vi "Main.vi"(11 "Module Admin":refnum<class "Delacor_lib_QMH_Module Admin.lvclass">) -> ()   [LabVIEW 2024, in "ProductControl.lvlib"]
doc: "This template is based off of the Queued Message Handler design pattern and the Queued Message Handler project template that ships with LabVIEW.\n\nThe main difference is that the queue is private to this module and communication between modules is performed via Broadcast and Request events.\n\nRequest events are wrapped in public API methods and are handled in the Event Handling Loop (EHL) of this VI. Any module can register for Broadcast events sent by this module. The EHL generates messages based on user interface actions.\n\nThe Message Handling Loop (MHL) processes messages generated by the EHL, or by other messages. The messages are string values, so new messages can be added easily to the Message Cases case structure in the MHL. Each message cluster can also provide an optional value for Message Data, which is a variant that can be converted to whatever message-specific data is required.\n_____\nBased on DQMH Dev Tools: Project Template 7.1.0.1503."
uses:
  ProductControl.lvlib
  <vilib>/Delacor/Delacor QMH/Libraries/Module Admin_class/Delacor_lib_QMH_Module Admin.lvclass
  Module Data--cluster.ctl
  Stop Argument--cluster.ctl
  <vilib>/Delacor/Delacor QMH/Libraries/Message Queue_class/Delacor_lib_QMH_Message Queue.lvclass/Delacor_lib_QMH_Message Queue.ctl
  <vilib>/Delacor/Delacor QMH/Libraries/Module Admin_class/Delacor_lib_QMH_Module Admin.lvclass/Delacor_lib_QMH_Module Admin.ctl
  Draw FP in Subpanel Argument--cluster.ctl
  Remove From Subpanel Argument--cluster.ctl
  Vender Producto Argument--cluster.ctl
  <vilib>/Delacor/Delacor QMH/Libraries/Message Queue_class/Delacor_lib_QMH_Enqueue Message (Single).vi
  <vilib>/Delacor/Delacor QMH/Libraries/Module Admin_class/Delacor_lib_QMH_Get External Launch.vi
  <vilib>/Delacor/Delacor QMH/Libraries/Message Queue_class/Delacor_lib_QMH_Message Queue.lvclass
panel:
  in  "Productos":i32(listbox)
  out "error out":errorcluster
  out "Status":string
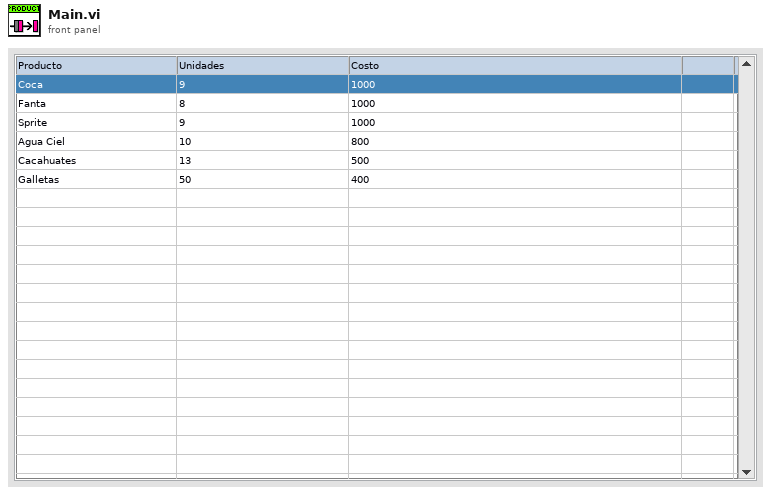
[diagram p1: front panel]
types:
  T1 = typedef "ProductControl.lvlib/Request Events--cluster.ctl" = cluster{"Stop Module":refnum<user-event>, "Show Panel":refnum<user-event>, "Hide Panel":refnum<user-event>, "Get Module Execution Status":refnum<user-event>, "Show Diagram":refnum<user-event>, "Draw FP in Subpanel":refnum<user-event>, "Remove From Subpanel":refnum<user-event>, "Vender Producto":refnum<user-event>}
  T2 = typedef "ProductControl.lvlib/Module Data--cluster.ctl" = cluster{"Status":string, "Sub Panel":refnum<vi>}
  T3 = enum32{"invalid lock state", "Not Locked", "Locked (No Password)", "Password-protected"}
  T4 = typedef "ProductControl.lvlib/Stop Argument--cluster.ctl" = cluster{"Origin":string, "Exit via Stop Module Req?":bool, "Wait for Module to stop?":bool}
  T5 = typedef "ProductControl.lvlib/Draw FP in Subpanel Argument--cluster.ctl" = cluster{"Sub Panel":refnum<vi>}
  T6 = typedef "ProductControl.lvlib/Remove From Subpanel Argument--cluster.ctl" = cluster{"Boolean":bool}
  T7 = typedef "ProductControl.lvlib/Vender Producto Argument--cluster.ctl" = cluster{"Nombre Producto":string}
  T8 = enum32{"Invalid", "Standard", "Closed", "Hidden", "Minimized", "Maximized"}
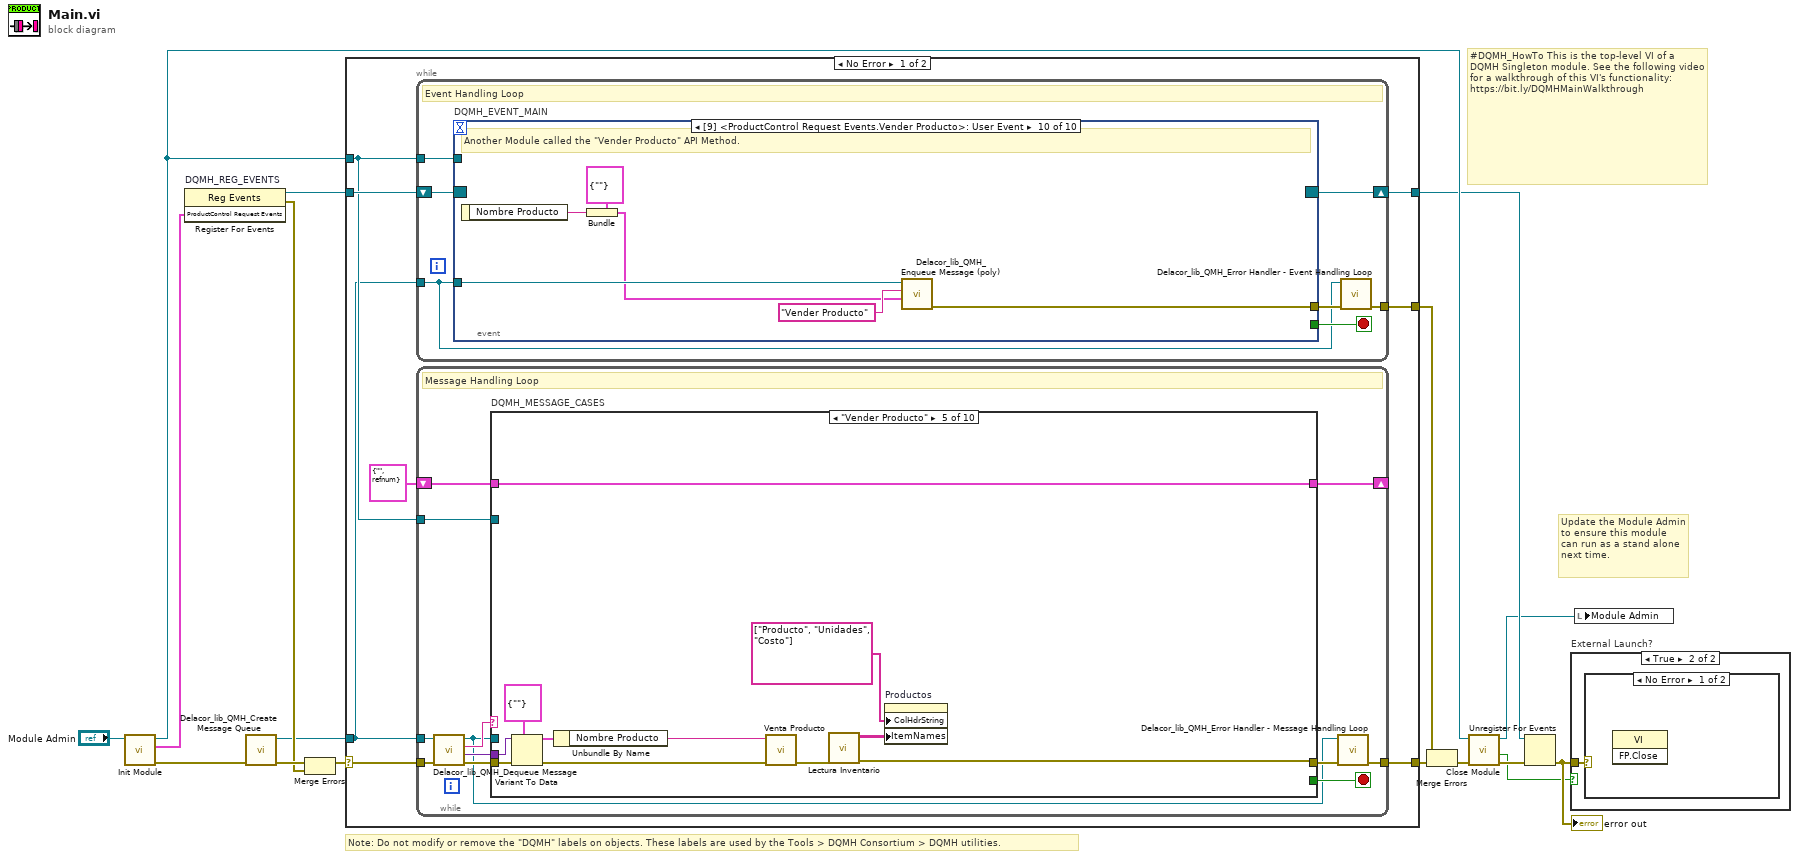
[diagram p0: block diagram]
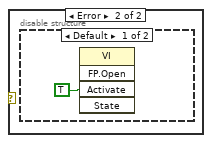
[diagram p3: hidden frame]
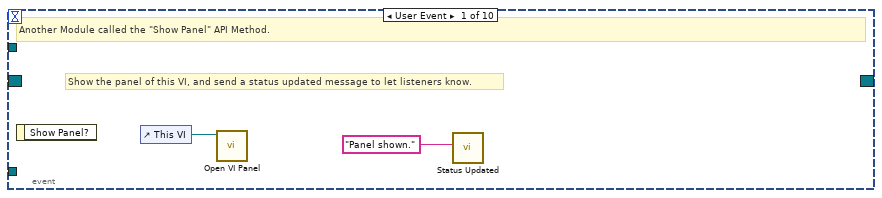
[diagram p5: hidden frame]
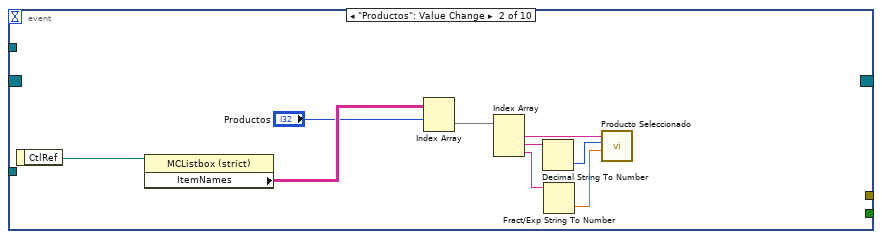
[diagram p6: hidden frame]
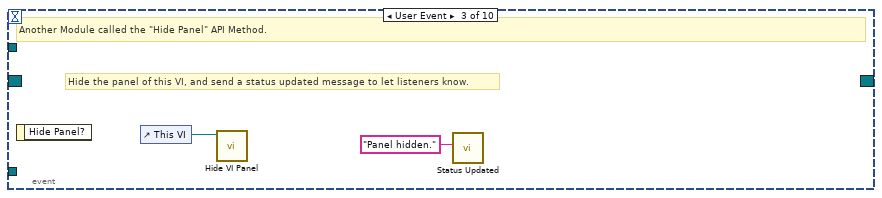
[diagram p7: hidden frame]
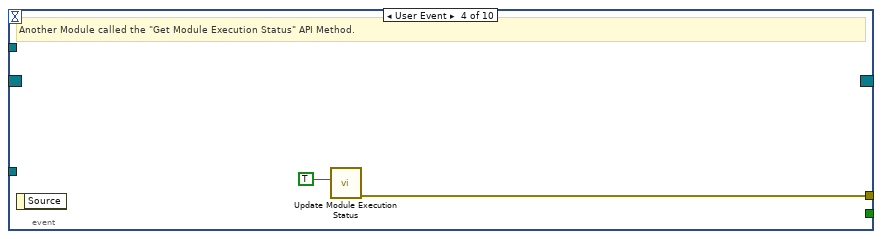
[diagram p8: hidden frame]
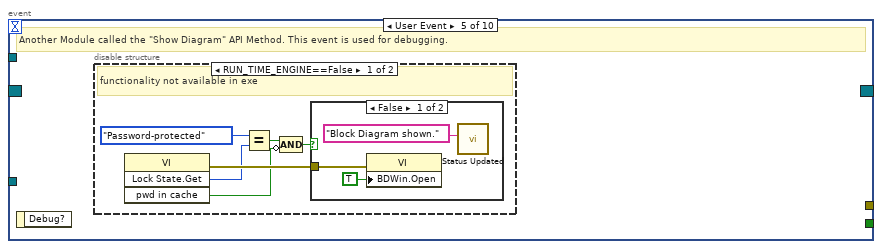
[diagram p9: hidden frame]
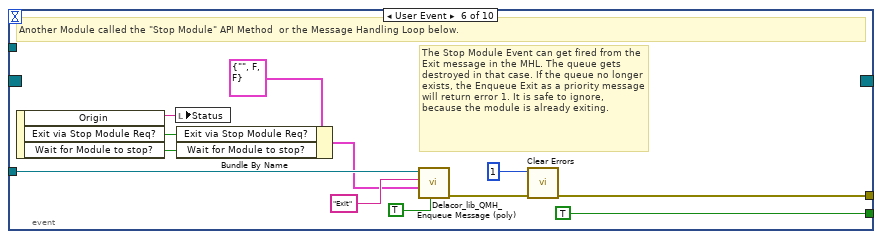
[diagram p12: hidden frame]
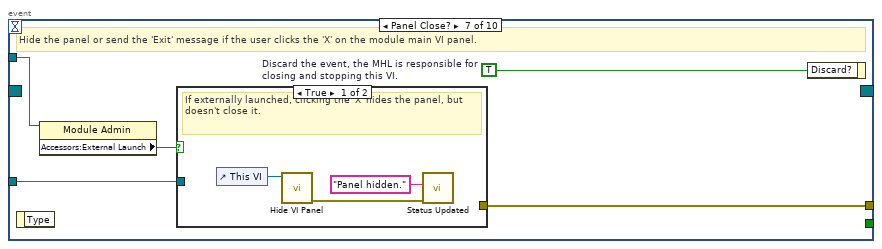
[diagram p13: hidden frame]
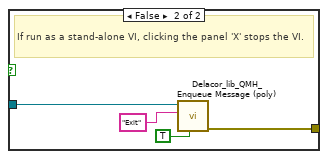
[diagram p14: hidden frame]
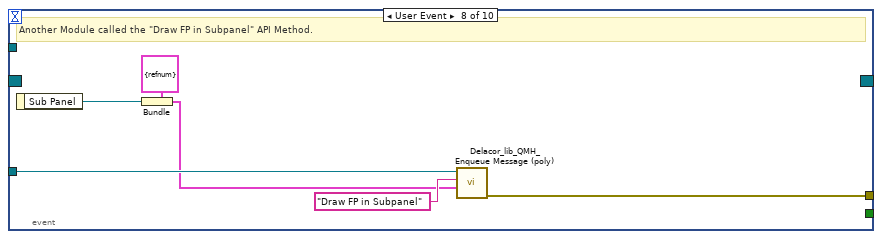
[diagram p15: hidden frame]
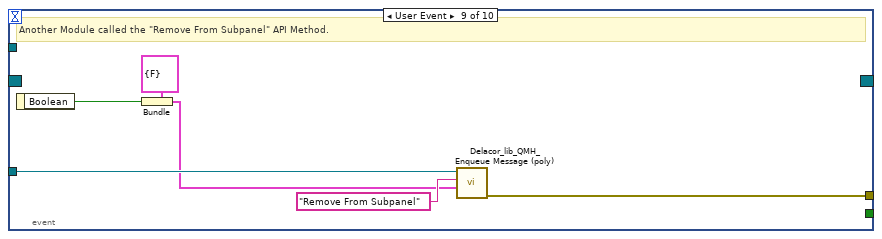
[diagram p16: hidden frame]
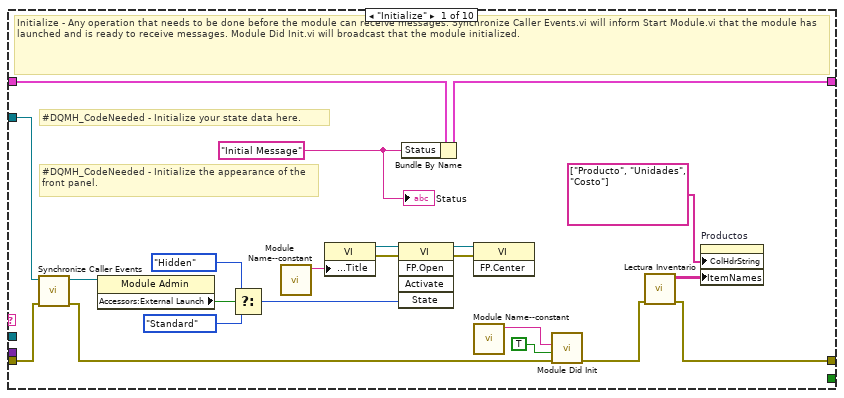
[diagram p17: hidden frame]
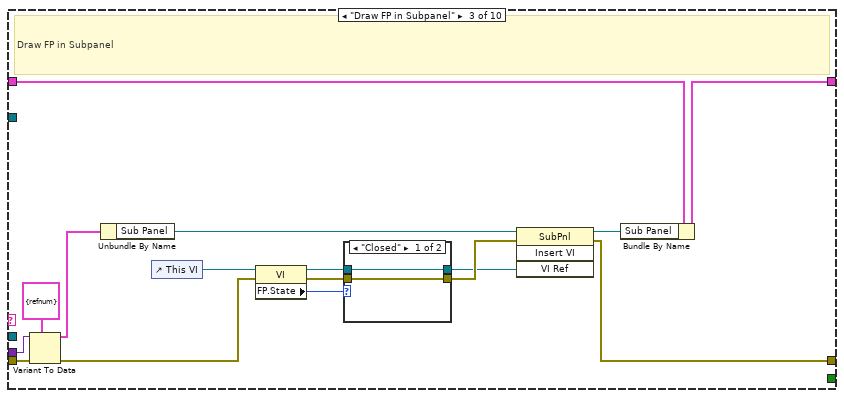
[diagram p19: hidden frame]
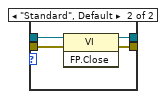
[diagram p20: hidden frame]
diagram:
  # "#DQMH_HowTo This is the top-level VI of a DQMH Singleton module. See the following video for a walkthrough of this VI's functionality: https://bit.ly/DQMHMainWalkthrough"
  # "Note: Do not modify or remove the \"DQMH\" labels on objects. These labels are used by the Tools > DQMH Consortium > DQMH utilities."
  # "Update the Module Admin to ensure this module can run as a stand alone next time."
  n1 = call "Init Module.vi"("Singleton Module Admin in"="Module Admin") -> ("error out"=w16:errorcluster, "ProductControl Request Events"=w5:T1, "Singleton Module Admin out"=w8:refnum<class "Delacor_lib_QMH_Module Admin.lvclass">)  [unwired: 8 in]
  n2 = register-events "DQMH_REG_EVENTS"(w5) -> (reference out=w6:refnum<event-registration>, error out=w9:errorcluster)  [unwired: 2 in]
  n3 = call <vilib>:"Delacor_lib_QMH_Create Message Queue.vi"("error in"=w16) -> ("error out"=w11:errorcluster, "Message Queue"=w4:refnum<class "Delacor_lib_QMH_Message Queue.lvclass">)  [unwired: 9 in]
  n4 = Merge Errors(w11, w9) -> (w10:errorcluster)
  n5 = case shown="No Error" w10 {
    selector: w10 -> [w23 w241]
    tunnel: [w25 w240] -> w17
    tunnel: [w22 w239] -> w7
    tunnel: w6 -> [w20 w239]
    tunnel: w4 -> [w18 w234]
    tunnel: [w24 _] -> w14
    tunnel: w8 -> [w19 w235]
    frame No Error {
      n6 = while {
        tunnel: w18 -> [w26]
        shift-right: [w29] -> w22
        shift-left: w20 -> [w30]
        tunnel: [w31] -> w24
        tunnel: w19 -> [w27]
        stop <- w28 stop-if-true
        # "Event Handling Loop"
        n7 = event "DQMH_EVENT_MAIN" shown="[9] <ProductControl Request Events.Vender Producto>: User Event" {
          selector: w30 -> [_ _ _ _ _ _ _ _ _ _]
          dyn-events: [_ _ _ _ _ _ _ _ _ _] -> w29
          timeout: _ -> [_ _ _ _ _ _ _ _ _ _]
          tunnel: [_ _ _ _ _ TRUE ("Discard?") _ _ _ _] -> w28
          tunnel: w26 -> [_ _ _ _ _ w64 w71 w85 w91 w97]
          tunnel: [_ _ _ w47 _ w67 w73 w86 w92 w98] -> w32
          tunnel: w27 -> [_ _ _ _ _ _ w70 _ _ _]
          event User Event {
            # "Show the panel of this VI, and send a status updated message to let listeners know."
            # "Another Module called the \"Show Panel\" API Method."
            n8 = event-data() -> ()  [unwired: 1 in, 1 out]
            n9 = control-ref of="This VI"() -> (w34:refnum<vi>)
            n10 = call "Open VI Panel.vi"("VI"=w34) -> ()  [unwired: 10 in, 1 out]
            n11 = call "Status Updated.vi"("Status"="Panel shown." ("format string")) -> ()  [unwired: 10 in, 1 out]
          }
          event "Productos": Value Change {
            n12 = event-data() -> ("CtlRef"=w43:refnum<vi>)  [unwired: 1 in]
            n13 = property class="MCListbox (strict)"(reference=w43) -> ("ItemNames"=w42:string[][])  [unwired: 1 in, 2 out]
            n14 = Index Array(array=w42, index (row)="Productos") -> (element=w40:string[])  [unwired: 1 in]
            n15 = Index Array(array=w40) -> (element #1=w39:string, element #2=w38:string, element #3=w36:string)  [unwired: 3 in]
            n16 = Decimal String To Number(string=w38) -> (number=w37:i32)  [unwired: 2 in, 1 out]
            n17 = Fract/Exp String To Number(string=w36) -> (number=w35:dbl)  [unwired: 3 in, 1 out]
            n18 = call "Producto Seleccionado.vi"("Costo"=w35, "Unidades"=w37, "Nombre Producto"=w39) -> ()  [unwired: 8 in, 1 out]
          }
          event User Event {
            # "Hide the panel of this VI, and send a status updated message to let listeners know."
            # "Another Module called the \"Hide Panel\" API Method."
            n19 = event-data() -> ()  [unwired: 1 in, 1 out]
            n20 = control-ref of="This VI"() -> (w45:refnum<vi>)
            n21 = call "Hide VI Panel.vi"("VI"=w45) -> ()  [unwired: 10 in, 1 out]
            n22 = call "Status Updated.vi"("Status"="Panel hidden." ("format string")) -> ()  [unwired: 10 in, 1 out]
          }
          event User Event {
            # "Another Module called the \"Get Module Execution Status\" API Method."
            n23 = event-data() -> ()  [unwired: 1 in, 1 out]
            n24 = call "Update Module Execution Status.vi"("Running?"=TRUE) -> ("error out"=w47:errorcluster)  [unwired: 10 in]
          }
          event User Event {
            # "Another Module called the \"Show Diagram\" API Method. This event is used for debugging."
            n25 = event-data() -> ()  [unwired: 1 in, 1 out]
            n26 = disable-structure shown="RUN_TIME_ENGINE==False" {
              frame condition #0 (active) {
                # "functionality not available in exe"
                n27 = invoke on="Invoke Node" class="VI" method="Lock State.Get"() -> (error out=w53:errorcluster, "Get Lock State"=w52:T3, "pwd in cache"=w49:bool)  [unwired: 4 in, 1 out]
                n28 = Equal?(x=T3."Password-protected", y=w52) -> (x = y?=w50:bool)
                n29 = Compound Arithmetic op=AND(w50, invert w49) -> (w48:bool)
                n30 = case shown="False" w48 {
                  tunnel: w53 -> [w56 _]
                  frame False {
                    n31 = property on="Property Node" class="VI"(error in=w56, "BDWin.Open"=TRUE ("Block Diagram Window:Open")) -> ()  [unwired: 1 in, 2 out]
                    n32 = call "Status Updated.vi"("Status"="Block Diagram shown." ("format string")) -> ()  [unwired: 10 in, 1 out]
                  }
                  frame True {
                    # "Password-protected VI, and the password is not in the cache. Do not show the diagram."
                  }
                }
              }
              frame condition #1 {
              }
            }
          }
          event User Event {
            # "The Stop Module Event can get fired from the Exit message in the MHL. The queue gets destroyed in that case. If the queue no longer exists, the Enqueue Exit as a priority message will return error 1. It is safe to ignore, because the module is already exiting."
            # "Another Module called the \"Stop Module\" API Method  or the Message Handling Loop below."
            n33 = event-data() -> ("Origin"=w63:string, "Exit via Stop Module Req?"=w59:bool, "Wait for Module to stop?"=w58:bool)  [unwired: 1 in]
            n34 = local write "Status"(w63) -> ()
            n35 = Bundle By Name(cluster=T4 {"Origin"="", "Exit via Stop Module Req?"=FALSE, "Wait for Module to stop?"=FALSE} ("Stop Argument"), "Exit via Stop Module Req?"=w59, "Wait for Module to stop?"=w58) -> (w57:T4)
            n36 = call-poly <vilib>:"Delacor_lib_QMH_Enqueue Message (poly).vi"("Priority Message? (F)"=TRUE, "Message Data"=w57, "Message"="Exit", "Message Queue in"=w64) -> ("error out"=w68:errorcluster)  [unwired: 6 in, 1 out]
            n37 = call <vilib>:"Clear Errors.vi"("error in (no error)"=w68, "specific error code to clear (0: all)"=1) -> ("error out"=w67:errorcluster)  [unwired: 4 in, 1 out]
          }
          event Panel Close? {
            w72 = TRUE  # Discard the event, the MHL is responsible for closing and stopping this VI.
            # "Hide the panel or send the 'Exit' message if the user clicks the 'X' on the module main VI panel."
            n38 = event-data() -> ()  [unwired: 1 in, 1 out]
            n39 = property on="Property Node" class="Module Admin"(reference=w70) -> ("Accessors:External Launch"=w69:bool)  [unwired: 1 in, 2 out]
            n40 = case shown="True" w69 {
              tunnel: w71 -> [_ w79]
              tunnel: [_ w80] -> w73
              frame True {
                # "If externally launched, clicking the 'X' hides the panel, but doesn't close it."
                n41 = control-ref of="This VI"() -> (w75:refnum<vi>)
                n42 = call "Hide VI Panel.vi"("VI"=w75) -> ("error out"=w76:errorcluster)  [unwired: 10 in]
                n43 = call "Status Updated.vi"("error in"=w76, "Status"="Panel hidden." ("format string")) -> ()  [unwired: 9 in, 1 out]
              }
              frame False {
                # "If run as a stand-alone VI, clicking the panel 'X' stops the VI."
                n44 = call-poly <vilib>:"Delacor_lib_QMH_Enqueue Message (poly).vi"("Priority Message? (F)"=TRUE, "Message"="Exit", "Message Queue in"=w79) -> ("error out"=w80:errorcluster)  [unwired: 7 in, 1 out]
              }
            }
            n45 = event-data ("Event Filter Node")("Discard?"=w72) -> ()  [unwired: 1 in, 1 out]
          }
          event User Event {
            # "Another Module called the \"Draw FP in Subpanel\" API Method."
            n46 = event-data() -> ("Sub Panel"=w81:refnum<vi>)  [unwired: 1 in]
            n47 = Bundle(cluster=T5 {"Sub Panel"=refnum} ("Draw FP in Subpanel Argument"), "Sub Panel"=w81) -> (w82:T5)
            n48 = call-poly <vilib>:"Delacor_lib_QMH_Enqueue Message (poly).vi"("Message Data"=w82, "Message"="Draw FP in Subpanel", "Message Queue in"=w85) -> ("error out"=w86:errorcluster)  [unwired: 7 in, 1 out]
          }
          event User Event {
            # "Another Module called the \"Remove From Subpanel\" API Method."
            n49 = event-data() -> ("Boolean"=w87:bool)  [unwired: 1 in]
            n50 = Bundle(cluster=T6 {"Boolean"=FALSE} ("Remove From Subpanel Argument"), "Boolean"=w87) -> (w88:T6)
            n51 = call-poly <vilib>:"Delacor_lib_QMH_Enqueue Message (poly).vi"("Message Data"=w88, "Message"="Remove From Subpanel", "Message Queue in"=w91) -> ("error out"=w92:errorcluster)  [unwired: 7 in, 1 out]
          }
          event User Event {
            # "Another Module called the \"Vender Producto\" API Method."
            n52 = event-data() -> ("Nombre Producto"=w93:string)  [unwired: 1 in]
            n53 = Bundle(cluster=T7 {"Nombre Producto"=""} ("Vender Producto Argument"), "Nombre Producto"=w93) -> (w94:T7)
            n54 = call-poly <vilib>:"Delacor_lib_QMH_Enqueue Message (poly).vi"("Message Data"=w94, "Message"="Vender Producto", "Message Queue in"=w97) -> ("error out"=w98:errorcluster)  [unwired: 7 in, 1 out]
          }
        }
        n55 = call-dynamic "Delacor_lib_QMH_Error Handler - Event Handling Loop.vi"("error in"=w32, "Message Queue in"=w26) -> ("dup error in"=w31:errorcluster)  [unwired: 8 in, 1 out]
      }
      n56 = while {
        tunnel: w18 -> [w99]
        shift-right: [w105] -> _
        shift-left: T2 {"Status"="", "Sub Panel"=refnum} ("Data Cluster") -> [w106]
        tunnel: w23 -> [w110]
        tunnel: [w108] -> w25
        tunnel: w19 -> [w101]
        stop <- w104 stop-if-true
        # "Message Handling Loop"
        n57 = call-dynamic "Delacor_lib_QMH_Dequeue Message.vi"("error in"=w110, "Message Queue in"=w99) -> ("error out"=w109:errorcluster, "Message Data"=w102:variant, "Message"=w103:string, "Message Queue out"=w100:refnum<class "Delacor_lib_QMH_Message Queue.lvclass">)  [unwired: 6 in]
        n58 = case "DQMH_MESSAGE_CASES" shown="\"Vender Producto\"" w103 {
          selector: w103 -> [_ _ _ _ _ _ _ _ _ w229]
          tunnel: w100 -> [_ _ _ _ _ _ _ w193 w217 _]
          tunnel: w109 -> [w130 w134 w150 w168 w185 w188 w190 w201 w223 w232]
          tunnel: [w127 w134 w149 w166 w182 w187 w190 w197 w218 w233] -> w107
          tunnel: w106 -> [w118 w133 w145 w162 w181 w186 w189 w195 w209 w230]
          tunnel: [w117 w133 w141 w159 w181 w186 w189 w195 w209 w230] -> w105
          tunnel: [_ _ _ _ _ _ _ _ w216 _] -> w104
          tunnel: w102 -> [_ _ w144 w165 w180 _ _ w194 w215 _]
          tunnel: w101 -> [w119 _ _ _ _ _ _ w192 w210 _]
          frame "Initialize" {
            w113 = "Initial Message" ("Initial Message")
            # "#DQMH_CodeNeeded - Initialize the appearance of the front panel."
            # "#DQMH_CodeNeeded - Initialize your state data here."
            # "Initialize - Any operation that needs to be done before the module can receive messages. Synchronize Caller Events.vi will inform Start Module.vi that the module has launched and is ready to receive messages. Module Did Init.vi will broadcast that the module initialized."
            n59 = call "Synchronize Caller Events.vi"("error in"=w130, "Singleton Module Admin in"=w119) -> ("error out"=w129:errorcluster, "Singleton Module Admin out"=w114:refnum<class "Delacor_lib_QMH_Module Admin.lvclass">)  [unwired: 8 in]
            n60 = property on="Property Node" class="Module Admin"(reference=w114) -> ("Accessors:External Launch"=w123:bool)  [unwired: 1 in, 2 out]
            n61 = Select(t=T8."Hidden" ("State"), s=w123, f=T8."Standard" ("State")) -> (s? t:f=w120:T8)
            n62 = call "Module Name--constant.vi"() -> ("Module Name"=w126:string)  [unwired: 11 in]
            n63 = property on="Property Node" class="VI"("Front Panel.Title"=w126) -> (reference out=w125:refnum<vi>, error out=w132:errorcluster)  [unwired: 2 in]
            n64 = invoke on="Invoke Node" class="VI" method="FP.Open"(reference=w125, error in=w132, "State"=w120) -> (reference out=w124:refnum<vi>, error out=w131:errorcluster)  [unwired: 2 in, 3 out]
            n65 = Bundle By Name(cluster=w118, "Status"=w113) -> (w117:T2)
            n66 = invoke on="Invoke Node" class="VI" method="FP.Center"(reference=w124, error in=w131) -> ()  [unwired: 1 in, 3 out]
            n67 = call "Module Name--constant.vi"() -> ("Module Name"=w115:string)  [unwired: 11 in]
            n68 = call "Module Did Init.vi"("error in"=w129, "Initialized?"=TRUE, "Origin"=w115) -> ("error out"=w128:errorcluster)  [unwired: 8 in]
            n69 = call "Lectura Inventario.vi"("error in"=w128) -> ("error out"=w127:errorcluster, "Inventario"=w112:string[][])  [unwired: 9 in]
            n70 = property on="Productos" class="MCListbox (strict)"("ColHdrString"=string[] ["Producto", "Unidades", "Costo"] ("Column Header Strings[]"), "ItemNames"=w112) -> ()  [unwired: 2 in, 2 out]
            "Status" <- w113
          }
          frame "---Module Specific---" {
            # "Separator -- The following cases handle messages specific to this Module."
          }
          frame "Draw FP in Subpanel" {
            # "Draw FP in Subpanel"
            n71 = Variant To Data(error in=w150, type=T5 {"Sub Panel"=refnum} ("Draw FP in Subpanel Argument"), Variant=w144) -> (data=w142:T5, error out=w148:errorcluster)
            n72 = Unbundle By Name(w142) -> ("Sub Panel"=w140:refnum<vi>)
            n73 = control-ref of="This VI"() -> (w137:refnum<vi>)
            n74 = property class="VI"(reference=w137, error in=w148) -> (reference out=w136:refnum<vi>, error out=w146:errorcluster, "FP.State"=w135:T8)
            n75 = case shown="\"Closed\"" w135 {
              tunnel: [w151 w154] -> w138
              tunnel: [w152 w156] -> w147
              tunnel: w146 -> [w152 w155]
              tunnel: w136 -> [w151 w153]
              frame "Closed" {
              }
              frame "Standard", Default {
                n76 = invoke class="VI" method="FP.Close"(reference=w153, error in=w155) -> (reference out=w154:refnum<vi>, error out=w156:errorcluster)  [unwired: 1 in, 1 out]
              }
            }
            n77 = invoke class="SubPnl" method="Insert VI"(reference=w140, error in=w147, "VI Ref"=w138) -> (reference out=w139:refnum<vi>, error out=w149:errorcluster)  [unwired: 1 in, 2 out]
            n78 = Bundle By Name(cluster=w145, "Sub Panel"=w139) -> (w141:T2)
          }
          frame "Remove From Subpanel" {
            # "Remove From Subpanel"
            n79 = Variant To Data(error in=w168, type=T6 {"Boolean"=FALSE} ("Remove From Subpanel Argument"), Variant=w165) -> (data=w163:T6, error out=w167:errorcluster)
            n80 = Unbundle By Name(w163) -> ()  [unwired: 1 out]
            n81 = Unbundle By Name(w162) -> ("Sub Panel"=w161:refnum<vi>)
            n82 = Not A Number/Path/Refnum?(number/path/refnum=w161) -> (NaN/Path/Refnum?=w160:bool)
            n83 = case shown="True" w160 {
              tunnel: w167 -> [w172 w174]
              tunnel: [w171 w174] -> w166
              tunnel: w161 -> [w170 _]
              tunnel: ["Module Removed from Subpanel" "This module has not been inserted into the subpanel"] -> w157
              frame False {
                n84 = invoke class="SubPnl" method="Remove VI"(reference=w170, error in=w172) -> (error out=w171:errorcluster)  [unwired: 1 in, 2 out]
              }
              frame True {
              }
            }
            n85 = Bundle By Name(cluster=w162, "Sub Panel"=refnum<vi> refnum) -> (w159:T2)
            n86 = call "Status Updated.vi"("Status"=w157) -> ()  [unwired: 10 in, 1 out]
          }
          frame "Vender Producto" {
            n87 = Variant To Data(error in=w185, type=T7 {"Nombre Producto"=""} ("Vender Producto Argument"), Variant=w180) -> (data=w178:T7, error out=w184:errorcluster)
            n88 = Unbundle By Name(w178) -> ("Nombre Producto"=w177:string)
            n89 = call "Venta Producto.vi"("error in"=w184, "Nombre Producto"=w177) -> ("error out"=w183:errorcluster)  [unwired: 9 in]
            n90 = call "Lectura Inventario.vi"("error in"=w183) -> ("error out"=w182:errorcluster, "Inventario"=w176:string[][])  [unwired: 9 in]
            n91 = property on="Productos" class="MCListbox (strict)"("ColHdrString"=string[] ["Producto", "Unidades", "Costo"] ("Column Header Strings[]"), "ItemNames"=w176) -> ()  [unwired: 2 in, 2 out]
          }
          frame "---Copy This Frame---" {
            # "Duplicate this frame when creating new messages.  Change this comment in the duplicated frame to describe this message."
            n92 = Merge Errors(w188) -> (w187:errorcluster)
          }
          frame "---Exit and Error Handling---" {
            # "Separator - The following cases handle errors and exit messages."
          }
          frame "Error" {
            # "#DQMH_CodeRecommended - If the module is running in standalone mode (External Launch = FALSE), this code will pop up an error dialog and call the 'Exit' message if an error occurs. Add more fine-grained error management here."
            # "Error - Check the error message data and respond accordingly. This message is sent by the \"Error Handler\" VIs at the end of each loop in this application."
            n93 = property on="Property Node" class="Module Admin"(reference=w192) -> ("Accessors:External Launch"=w191:bool)  [unwired: 1 in, 2 out]
            n94 = Variant To Data(error in=w201, type=errorcluster {"status"=FALSE, "code"=0, "source"=""} ("error constant"), Variant=w194) -> (data=w196:errorcluster, error out=w199:errorcluster)
            n95 = local write "error out"(w196) -> ()
            n96 = call "Error Reported.vi"("Error"=w196) -> ()  [unwired: 10 in, 1 out]
            n97 = case shown="False" w191 {
              tunnel: [w206 _] -> w198
              tunnel: w193 -> [w204 _]
              tunnel: w196 -> [w205 _]
              frame False {
                n98 = disable-structure shown="Default" {
                  disable-tunnel: w205 -> [w207 _]
                  frame condition #0 (active) {
                    # "If the module is running standalone, then pop up an error dialog and call the \"Exit\" message."
                    n99 = call <vilib>:"Simple Error Handler.vi"("error in (no error)"=w207) -> ()  [unwired: 4 in, 5 out]
                  }
                  frame condition #1 {
                    # "To prevent the Simple Error Handler VI from being loaded (e.g. when deploying to a Real-Time target), add the Conditional Disable Symbol \"DQMH_Disable_SEH\" to your project and set it to TRUE."
                  }
                }
                n100 = call-poly <vilib>:"Delacor_lib_QMH_Enqueue Message (poly).vi"("Priority Message? (F)"=TRUE, "Message"="Exit", "Message Queue in"=w204) -> ("error out"=w206:errorcluster)  [unwired: 7 in, 1 out]
              }
              frame True {
                # "If the module was launched externally, calling the Error Reported broadcast VI is the only action performed by the \"Error\" message. The module's caller can then process the error appropriately."
              }
            }
            n101 = Merge Errors(w199, w198) -> (w197:errorcluster)
          }
          frame "Exit" {
            w214 = 91  # 91: not all Exit messages will have an argument
            w216 = TRUE  # Stop the VI
            # "Release the message queue reference"
            # "#DQMH_CodeNeeded - Add any required cleanup code here."
            # "Exit - Exit the application."
            n102 = Variant To Data(error in=w223, type=T4 {"Origin"="", "Exit via Stop Module Req?"=FALSE, "Wait for Module to stop?"=FALSE} ("Stop Argument"), Variant=w215) -> (data=w212:T4, error out=w220:errorcluster)
            n103 = call <vilib>:"Clear Errors.vi"("error in (no error)"=w220, "specific error code to clear (0: all)"=w214) -> ("error out"=w222:errorcluster)  [unwired: 4 in, 1 out]
            n104 = control-ref of="This VI"() -> (w211:refnum<vi>)
            n105 = call-dynamic "Delacor_lib_QMH_Release Message Queue.vi"("error in"=w222, "Message Queue"=w217) -> ("error out"=w221:errorcluster)  [unwired: 9 in]
            n106 = call "Handle Exit.vi"("Stop Argument"=w212, "Admin in"=w210, "VI reference"=w211) -> ("error out"=w219:errorcluster)  [unwired: 7 in, 1 out]
            n107 = Merge Errors(w221, w219) -> (w218:errorcluster)
            n108 = Unbundle By Name(w209) -> ("Sub Panel"=w208:refnum<vi>)
            n109 = call "Error Reported.vi"("Error"=w218) -> ()  [unwired: 10 in, 1 out]
            n110 = invoke class="SubPnl" method="Remove VI"(reference=w208) -> ()  [unwired: 2 in, 3 out]
          }
          frame Default {
            # "'Default' case only runs if there is a message that isn't defined in any of the other cases.  Output a programming error."
            n111 = call "Module Name--constant.vi"() -> ("Module Name"=w228:string)  [unwired: 11 in]
            n112 = Format Into String(format string="The invalid message string \"%s\" was received in the Message Handling Loop for module \"%s\".", w229, w228) -> (resulting string=w224:string)  [unwired: 2 in, 1 out]
            n113 = call <vilib>:"Error Cluster From Error Code.vi"("show call chain? (False)"=TRUE, "error message (\"\")"=w224, "error code (0)"=1) -> ("error out"=w231:errorcluster)  [unwired: 6 in]
            n114 = Merge Errors(w232, w231) -> (w233:errorcluster)
          }
        }
        n115 = call-dynamic "Delacor_lib_QMH_Error Handler - Message Handling Loop.vi"("error in"=w107, "Message Queue in"=w100) -> ("dup error in"=w108:errorcluster)  [unwired: 8 in, 1 out]
      }
    }
    frame Error {
      # "Synchronize Caller Events.vi will inform Start Module.vi that the module has launched and will let the code calling Start Module.vi register for broadcasts and would permit the caller receive the broadcast that an error occurred at launch time."
      n116 = call-dynamic "Delacor_lib_QMH_Release Message Queue.vi"("error in"=w241, "Message Queue"=w234) -> ("error out"=w240:errorcluster)  [unwired: 9 in]
      n117 = call "Synchronize Caller Events.vi"("Singleton Module Admin in"=w235) -> ("error out"=w242:errorcluster)  [unwired: 9 in, 1 out]
      n118 = call "Module Name--constant.vi"() -> ("Module Name"=w238:string)  [unwired: 11 in]
      n119 = Format Into String(format string="An error occurred during initialization. %s is no longer running.", w238) -> (resulting string=w236:string)  [unwired: 2 in, 1 out]
      n120 = Merge Errors(w240, w242) -> (w243:errorcluster)
      n121 = call "Error Reported.vi"("Additional Information"=w236, "Error"=w243) -> ()  [unwired: 9 in, 1 out]
    }
  }
  n122 = Merge Errors(w14, w17) -> (w13:errorcluster)
  n123 = call "Close Module.vi"("error in"=w13, "Module Admin in"=w8) -> ("error out"=w15:errorcluster, "External Launch"=w1:bool, "Module Admin out"=w2:refnum<class "Delacor_lib_QMH_Module Admin.lvclass">)  [unwired: 7 in]
  n124 = Unregister For Events(event registration refnum=w7, error in=w15) -> (error out=w12:errorcluster)
  "error out" <- w12
  n125 = case "External Launch?" shown="True" w1 {
    tunnel: w12 -> [_ w244]
    frame False {
    }
    frame True {
      n126 = case shown="No Error" w244 {
        frame No Error {
          n127 = invoke on="Invoke Node" class="VI" method="FP.Close"() -> ()  [unwired: 3 in, 3 out]
        }
        frame Error {
          n128 = disable-structure shown="Default" {
            frame condition #0 (active) {
              n129 = invoke class="VI" method="FP.Open"("Activate"=TRUE ("Activate?")) -> ()  [unwired: 4 in, 5 out]
            }
            frame condition #1 {
              # "Don't show panel on error if running inside a built EXE."
            }
          }
        }
      }
    }
  }
  n130 = local write "Module Admin"(w2) -> ()
